vi "Start - Stop Postions1.vi"(5 "New Status of Positions":bool[](array[boolean]), 7 "Rack Number":i16=1 min=1 max=16, 11 "System#":u8=1 min=1 max=16) -> ()   [LabVIEW 2021]
uses:
  Main Controls System v8.0/AutoAge Globals.vi
panel:
  out "At least 1 position\nhas started":bool
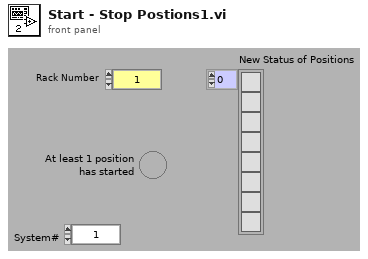
[diagram p1: front panel]
types:
  T1 = enum32{"existing file", "new file", "new or existing file", "existing dir", "new dir", "new or existing dir", "existing file (use LLBs)", "new file (use LLBs)", "new or existing file (use LLBs)", "new or existing file or directory (use LLBs)"}
  T2 = enum16{"open", "replace", "create", "open or create", "replace or create", "replace or create with confirmation"}
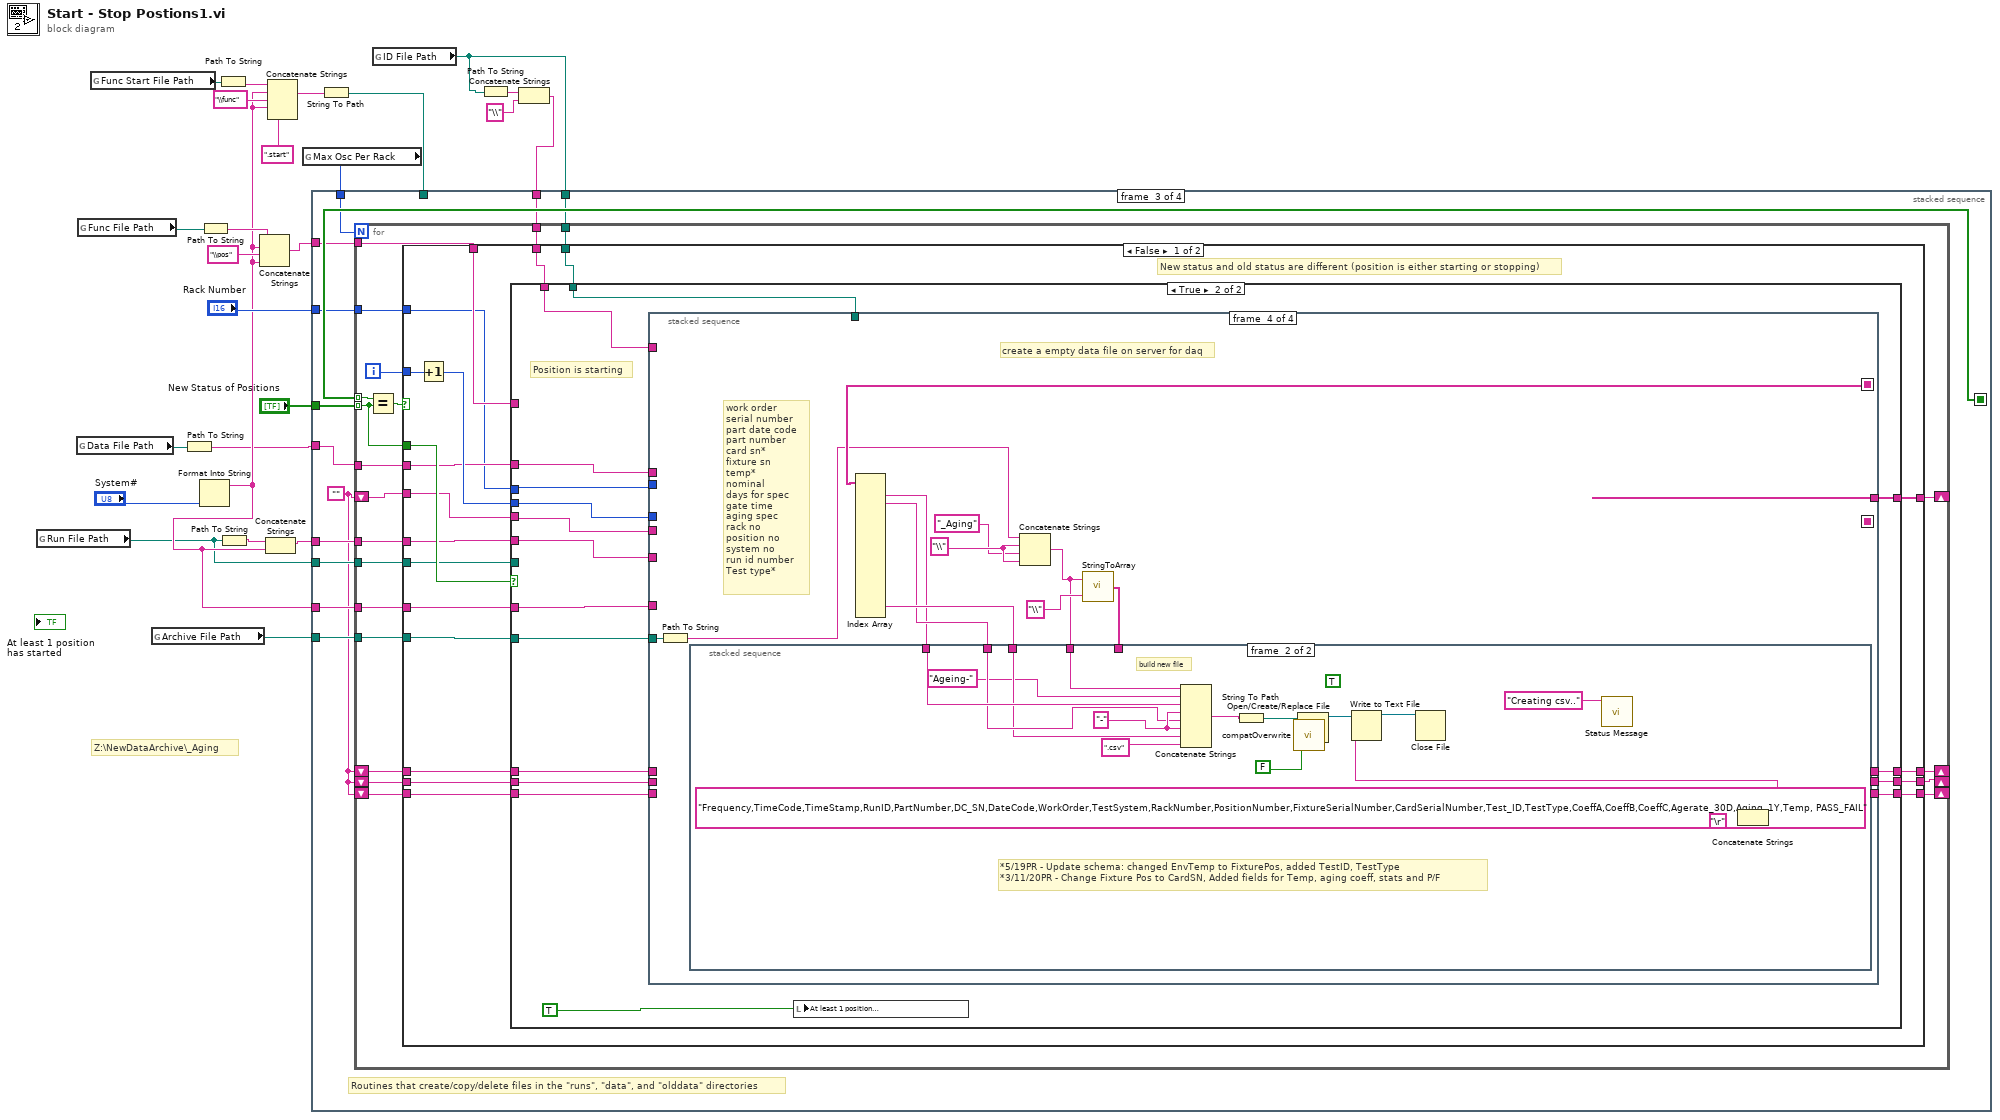
[diagram p0: block diagram]
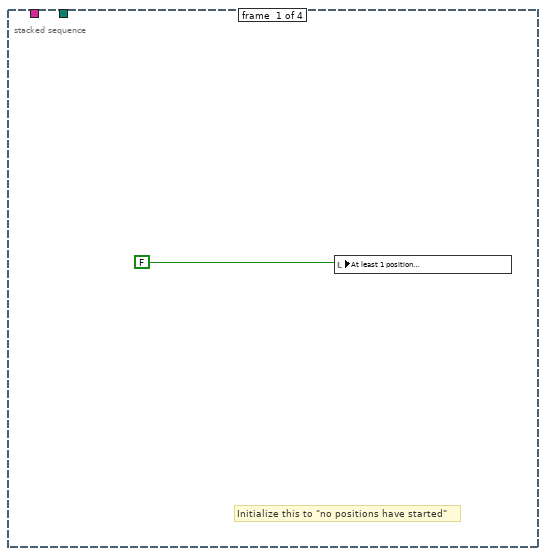
[diagram p2: hidden frame]
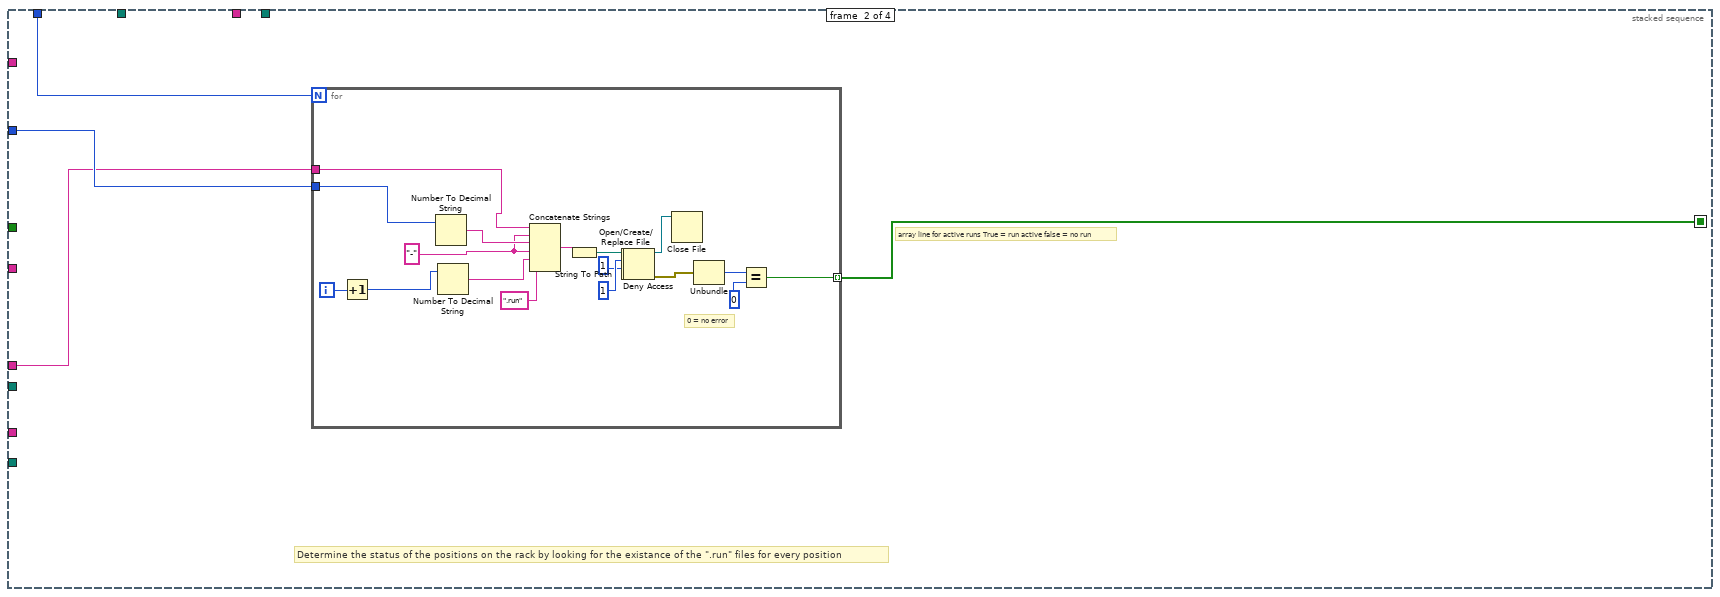
[diagram p3: hidden frame]
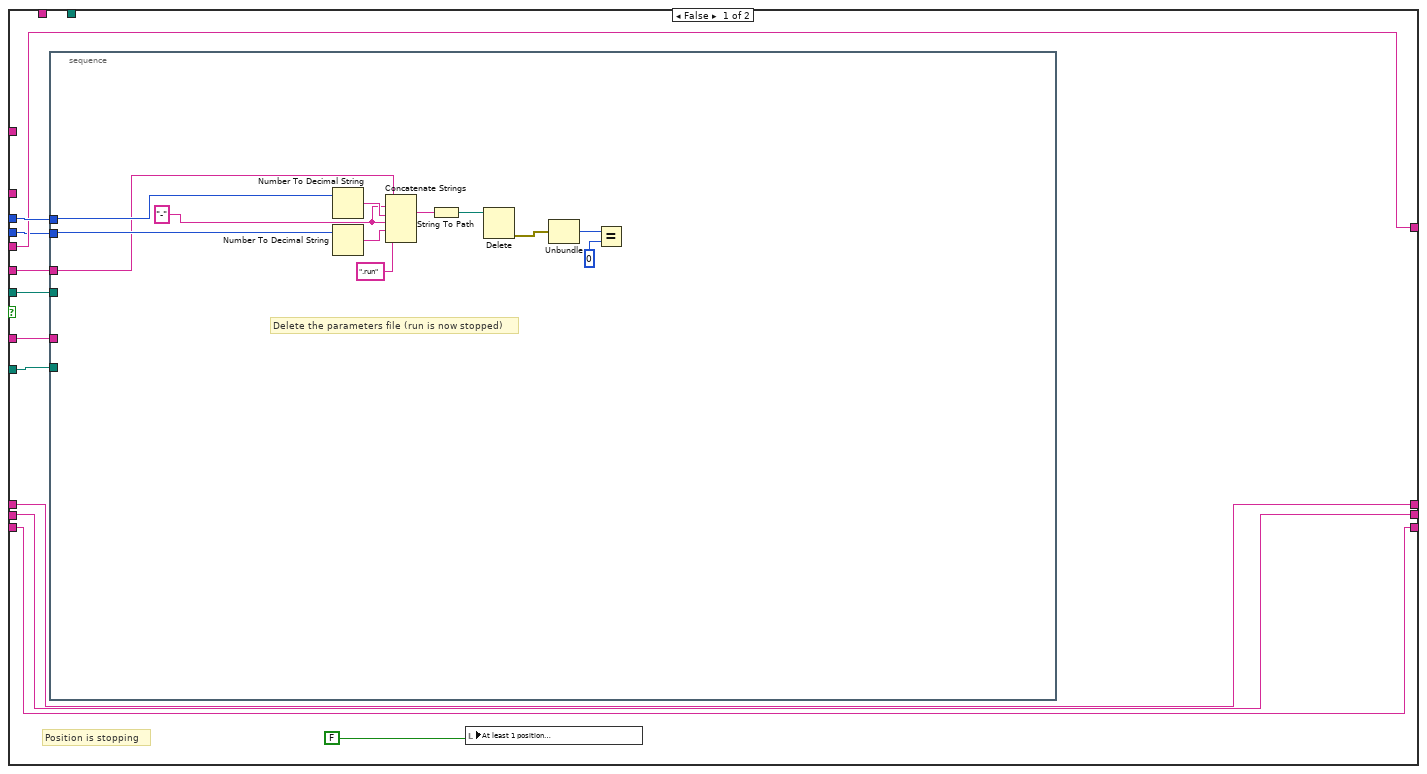
[diagram p4: hidden frame]
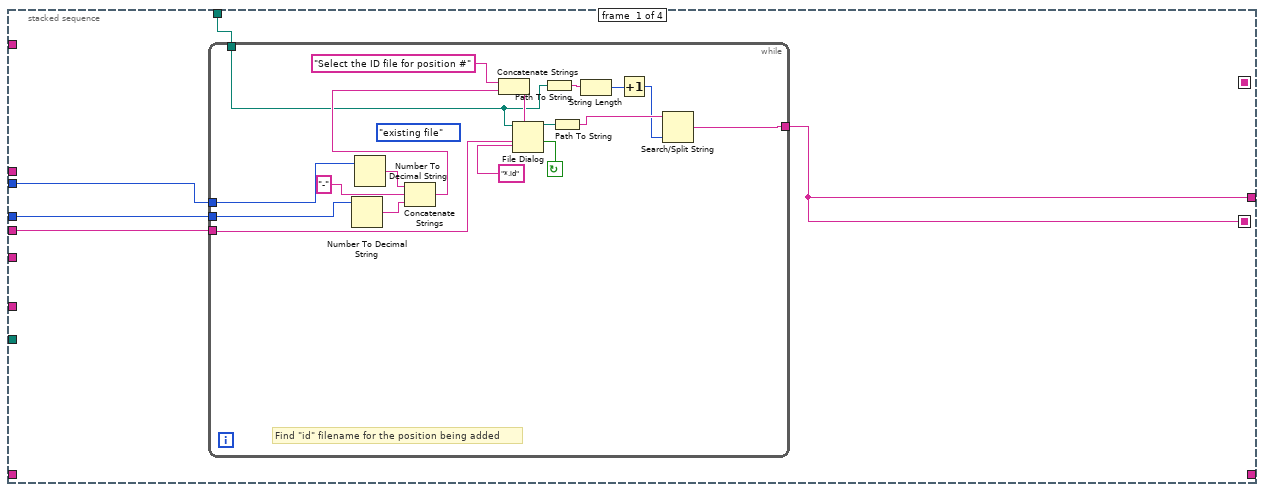
[diagram p5: hidden frame]
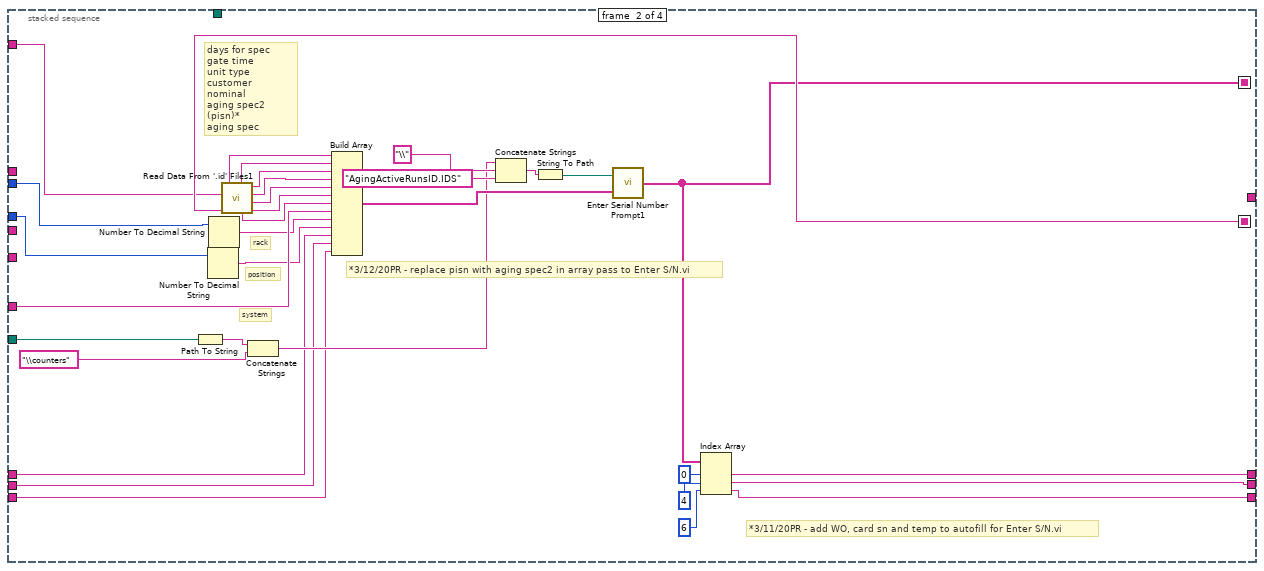
[diagram p6: hidden frame]
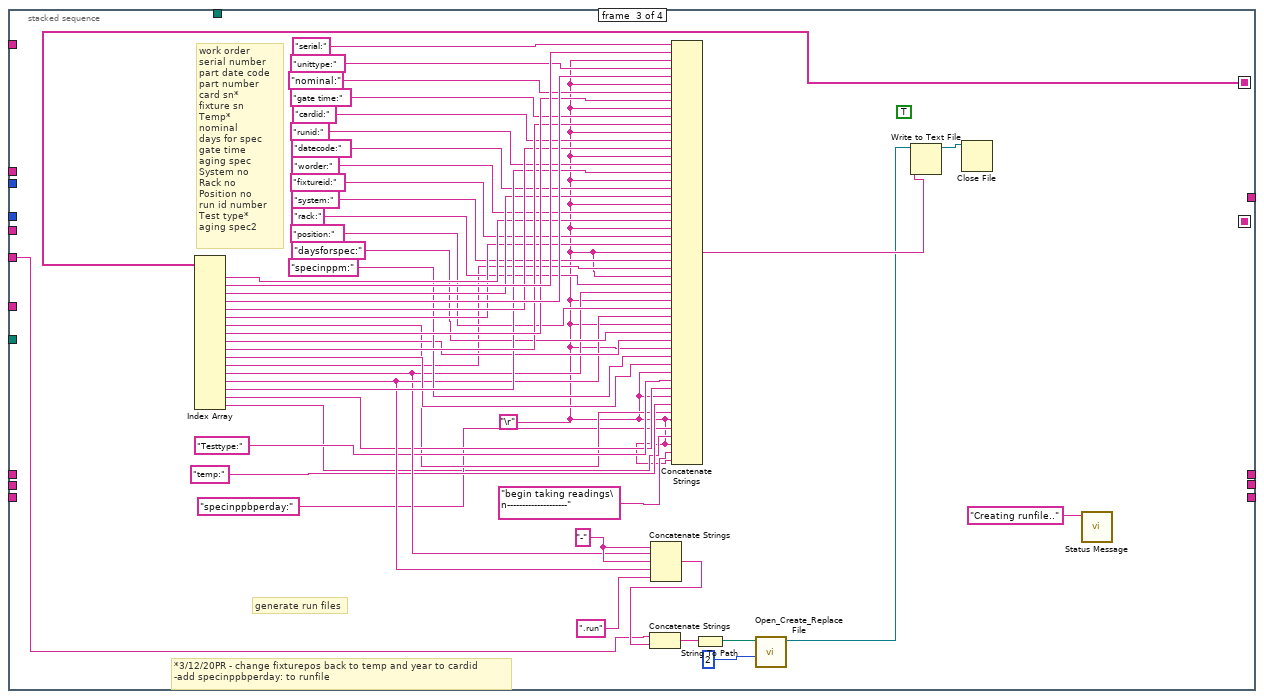
[diagram p7: hidden frame]
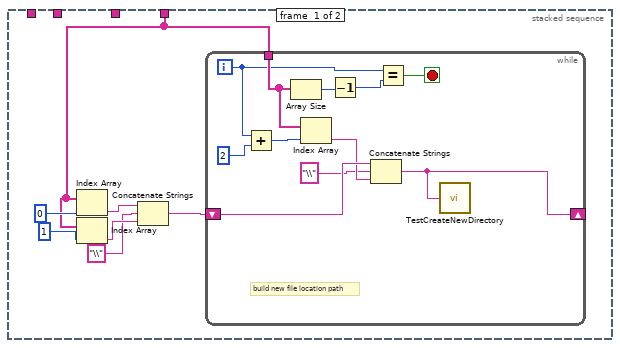
[diagram p8: hidden frame]
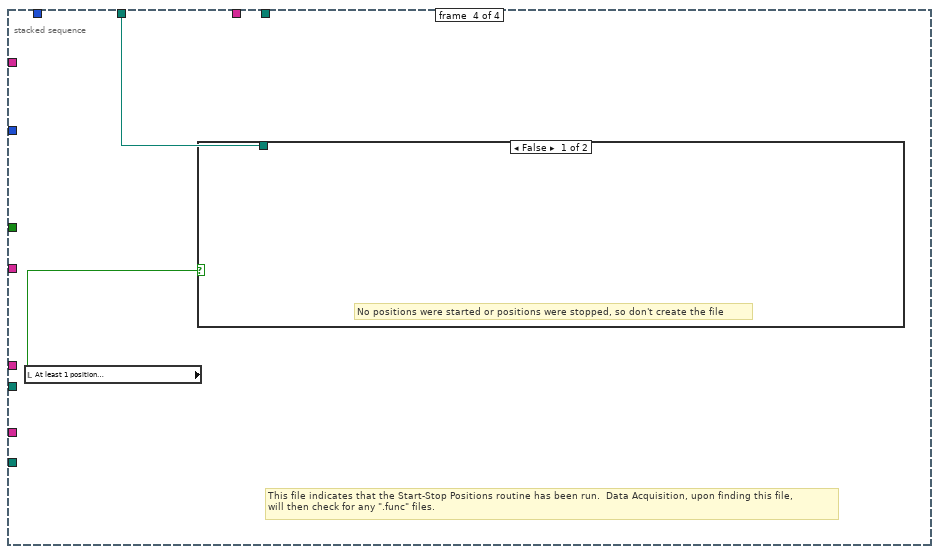
[diagram p10: hidden frame]
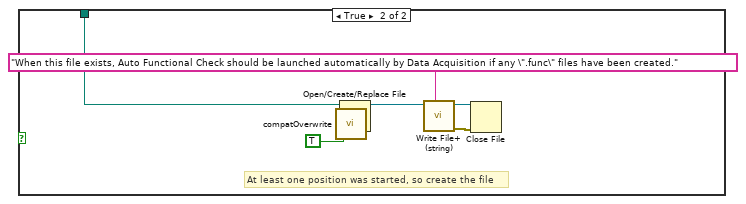
[diagram p11: hidden frame]
diagram:
  # "Z:\\NewDataArchive\\_Aging"
  n1 = global read "AutoAge Globals.vi" "Run File Path"() -> (w2:path)
  n2 = global read "AutoAge Globals.vi" "Data File Path"() -> (w15:path)
  n3 = global read "AutoAge Globals.vi" "Func File Path"() -> (w16:path)
  n4 = global read "AutoAge Globals.vi" "Func Start File Path"() -> (w17:path)
  n5 = global read "AutoAge Globals.vi" "Archive File Path"() -> (w14:path)
  n6 = Path To String(path=w15) -> (string=w1:string)
  n7 = Format Into String("System#") -> (resulting string=w3:string)  [unwired: 3 in, 1 out]
  n8 = Path To String(path=w16) -> (string=w21:string)
  n9 = Path To String(path=w17) -> (string=w8:string)
  n10 = Path To String(path=w2) -> (string=w22:string)
  n11 = Concatenate Strings(w21, w3, "\\pos" ("Substring"), w3) -> (w20:string)
  n12 = Concatenate Strings(w22, w3) -> (w23:string)
  n13 = Concatenate Strings(w8, w3, "\\func" ("Substring"), w3, ".start" ("Substring")) -> (w19:string)
  n14 = global read "AutoAge Globals.vi" "Max Osc Per Rack"() -> (w4:u16)
  n15 = String To Path(string=w19) -> (path=w18:path)
  n16 = global read "AutoAge Globals.vi" "ID File Path"() -> (w12:path)
  n17 = Path To String(path=w12) -> (string=w11:string)
  n18 = Concatenate Strings(w11, "\\" ("Substring")) -> (w9:string)
  n19 = stacked-sequence {
    seq-local: [_ w29 _ _] -> [_ _ w62 _]
    tunnel: "Rack Number" -> [_ w30 w54 _]
    tunnel: "New Status of Positions" -> [_ _ w61 _]
    tunnel: w9 -> [_ _ w59 _]
    tunnel: w23 -> [_ w27 w57 _]
    tunnel: w1 -> [_ _ w58 _]
    tunnel: w14 -> [_ _ w56 _]
    tunnel: w20 -> [_ _ w55 _]
    tunnel: w18 -> [_ _ _ w298]
    tunnel: w12 -> [_ _ w53 _]
    tunnel: w4 -> [_ w28 w60 _]
    tunnel: w3 -> [_ _ w52 _]
    tunnel: w2 -> [_ _ w51 _]
    frame #0 {
      # "Initialize this to \"no positions have started\""
      n20 = local write "At least 1 position\nhas started"(FALSE) -> ()
    }
    frame #1 {
      # "array line for active runs True = run active false = no run"
      # "Determine the status of the positions on the rack by looking for the existance of the \".run\" files for every position"
      n21 = for {
        N: w28 -> [_]
        tunnel: [w48] -> w29 mode=indexing
        tunnel: w30 -> [w38]
        tunnel: w27 -> [w33]
        i -> [w49]
        w34 = "-"
        # "0 = no error"
        n22 = Increment(x=w49) -> (x+1=w35:i32)
        n23 = Number To Decimal String(number=w38) -> (decimal integer string=w37:string)  [unwired: 1 in]
        n24 = Number To Decimal String(number=w35) -> (decimal integer string=w36:string)  [unwired: 1 in]
        n25 = Concatenate Strings(w33, w34, w37, w34, w36, ".run") -> (w47:string)
        n26 = String To Path(string=w47) -> (path=w46:path)
        n27 = Open/Create/Replace File(file path (use dialog)=w46, access (0:read/write)=1) -> (refnum out=w31:refnum<file>, error out=w32:errorcluster)  [unwired: 4 in, 1 out]
        n28 = Deny Access(4:w32, 6:1, 7:w31) -> (0:w43:errorcluster, 3:w40:refnum<file>)
        n29 = Close File(refnum=w40) -> ()  [unwired: 1 in, 2 out]
        n30 = Unbundle(w43) -> ("code"=w41:i32)  [unwired: 2 out]
        n31 = Equal?(x=w41, y=0) -> (x = y?=w48:bool)
      }
    }
    frame #2 {
      w50 = ""
      # "Routines that create/copy/delete files in the \"runs\", \"data\", and \"olddata\" directories"
      n32 = for {
        N: w60 -> [_]
        tunnel: w62 -> [w82] mode=indexing
        tunnel: w61 -> [w81] mode=indexing
        shift-right: [w78] -> _
        shift-left: w50 -> [w79]
        tunnel: w59 -> [w77]
        tunnel: w58 -> [w76]
        tunnel: w57 -> [w75]
        tunnel: w56 -> [w74]
        tunnel: w55 -> [w73]
        tunnel: w54 -> [w72]
        tunnel: w53 -> [w71]
        tunnel: w52 -> [w70]
        tunnel: w51 -> [w69]
        shift-right: [w68] -> _
        shift-left: w50 -> [w65]
        shift-right: [w67] -> _
        shift-left: w50 -> [w64]
        shift-right: [w66] -> _
        shift-left: w50 -> [w63]
        i -> [w80]
        n33 = Equal?(x=w82, y=w81) -> (x = y?=w83:bool)
        n34 = case shown="False" w83 {
          tunnel: w81 -> [w103 _]
          tunnel: w80 -> [w100 _]
          tunnel: w79 -> [w102 w297]
          tunnel: [w101 w297] -> w78
          tunnel: w77 -> [w98 _]
          tunnel: w76 -> [w97 _]
          tunnel: w75 -> [w96 _]
          tunnel: w74 -> [w95 _]
          tunnel: w73 -> [w94 _]
          tunnel: w72 -> [w93 _]
          tunnel: w71 -> [w92 _]
          tunnel: w70 -> [w91 _]
          tunnel: w69 -> [w90 _]
          tunnel: [w89 w296] -> w68
          tunnel: [w88 w295] -> w67
          tunnel: [w87 w294] -> w66
          tunnel: w65 -> [w86 w296]
          tunnel: w64 -> [w85 w295]
          tunnel: w63 -> [w84 w294]
          frame False {
            # "New status and old status are different (position is either starting or stopping)"
            n35 = Increment(x=w100) -> (x+1=w99:i32)
            n36 = case shown="True" w103 {
              tunnel: w93 -> [w114 w136]
              tunnel: w102 -> [w113 w143]
              tunnel: [w113 w142] -> w101
              tunnel: w99 -> [w112 w141]
              tunnel: w98 -> [_ w139]
              tunnel: w97 -> [_ w138]
              tunnel: w96 -> [w110 w137]
              tunnel: w95 -> [w109 w133]
              tunnel: w94 -> [_ _]
              tunnel: w92 -> [_ w135]
              tunnel: w91 -> [w108 w134]
              tunnel: w90 -> [w107 _]
              tunnel: [w106 w132] -> w89
              tunnel: [w105 w131] -> w88
              tunnel: [w104 w130] -> w87
              tunnel: w86 -> [w106 w129]
              tunnel: w85 -> [w105 w128]
              tunnel: w84 -> [w104 w127]
              frame False {
                # "Position is stopping"
                n37 = stacked-sequence {
                  tunnel: w114 -> [w118]
                  tunnel: w112 -> [w117]
                  tunnel: w110 -> [w115]
                  tunnel: w109 -> [_]
                  tunnel: w108 -> [_]
                  tunnel: w107 -> [_]
                  frame #0 {
                    w116 = "-"
                    # "Delete the parameters file (run is now stopped)"
                    n38 = Number To Decimal String(number=w118) -> (decimal integer string=w120:string)  [unwired: 1 in]
                    n39 = Number To Decimal String(number=w117) -> (decimal integer string=w119:string)  [unwired: 1 in]
                    n40 = Concatenate Strings(w115, w116, w120, w116, w119, ".run") -> (w126:string)
                    n41 = String To Path(string=w126) -> (path=w125:path)
                    n42 = Delete(path (use dialog)=w125) -> (error out=w123:errorcluster)  [unwired: 4 in, 2 out]
                    n43 = Unbundle(w123) -> ("code"=w124:i32)  [unwired: 2 out]
                    n44 = Equal?(x=w124, y=0) -> ()  [unwired: 1 out]
                  }
                }
                n45 = local write "At least 1 position\nhas started"(FALSE) -> ()
              }
              frame True {
                # "Position is starting"
                n46 = stacked-sequence {
                  seq-local: [w147 _ _ _] -> [_ w199 _ _]
                  seq-local: [_ w177 _ _] -> [_ _ w244 w258]
                  tunnel: w136 -> [w145 w190 _ _]
                  tunnel: w143 -> [w148 _ _ _]
                  tunnel: [w147 _ _ _] -> w142
                  tunnel: w141 -> [w146 w189 _ _]
                  tunnel: w139 -> [_ w198 _ _]
                  tunnel: w138 -> [_ _ _ _]
                  tunnel: w137 -> [_ _ w242 _]
                  tunnel: w135 -> [w144 _ _ _]
                  tunnel: w134 -> [_ w184 _ _]
                  tunnel: w133 -> [_ w181 _ w257]
                  tunnel: [_ w173 _ _] -> w132
                  tunnel: [_ w172 _ _] -> w131
                  tunnel: [_ w171 _ _] -> w130
                  tunnel: w129 -> [_ w170 _ _]
                  tunnel: w128 -> [_ w169 _ _]
                  tunnel: w127 -> [_ w168 _ _]
                  frame #0 {
                    n47 = while {
                      tunnel: w144 -> [w153]
                      tunnel: w146 -> [w158]
                      tunnel: w145 -> [w156]
                      tunnel: [w149] -> w147
                      tunnel: w148 -> [w165]
                      stop <- w166 continue-if-true
                      (unwired) T1."existing file" ("select mode (2)")
                      # "Find \"id\" filename for the position being added"
                      n48 = Number To Decimal String(number=w158) -> (decimal integer string=w160:string)  [unwired: 1 in]
                      n49 = Number To Decimal String(number=w156) -> (decimal integer string=w155:string)  [unwired: 1 in]
                      n50 = Concatenate Strings(w155, "-", w160) -> (w157:string)
                      n51 = Concatenate Strings("Select the ID file for position #" ("prompt"), w157) -> (w161:string)
                      n52 = File Dialog(6:"*.id" ("pattern"), 7:w161, 9:w165, 11:w153) -> (1:w166:bool, 3:w163:path)  [unwired: 3 in, 2 out]
                      n53 = Path To String(path=w153) -> (string=w152:string)
                      n54 = Path To String(path=w163) -> (string=w162:string)
                      n55 = String Length(string=w152) -> (length=w151:i32)
                      n56 = Increment(x=w151) -> (x+1=w150:i32)
                      n57 = Search/Split String(string=w162, offset (0)=w150) -> (match + rest of string=w149:string)  [unwired: 1 in, 2 out]
                    }
                  }
                  frame #1 {
                    # "*3/12/20PR - replace pisn with aging spec2 in array pass to Enter S/N.vi"
                    # "*3/11/20PR - add WO, card sn and temp to autofill for Enter S/N.vi"
                    # "system"
                    # "position"
                    # "rack"
                    # "days for spec\ngate time\nunit type\ncustomer\nnominal\naging spec2 (pisn)*\naging spec"
                    n58 = Path To String(path=w181) -> (string=w180:string)
                    n59 = Number To Decimal String(number=w189) -> (decimal integer string=w182:string)  [unwired: 1 in]
                    n60 = Number To Decimal String(number=w190) -> (decimal integer string=w183:string)  [unwired: 1 in]
                    n61 = call "Read Data From '.id' Files1.vi"("ID File Path"=w198, "ID Filename"=w199) -> ("# Days for Aging Spec"=w197:string, "Gate Time"=w196:string, "Aging Spec"=w192:string, "Unit Type"=w195:string, "Customer"=w194:string, "Nominal Frequency"=w193:string, "Aging Spec 2"=w167:string)  [unwired: 1 out]
                    n62 = Concatenate Strings(w180, "\\counters") -> (w178:string)
                    n63 = Build Array(w197, w196, w195, w194, w193, w167, w192, w184, w183, w182, w170, w169, w168) -> (w191:string[])
                    n64 = Concatenate Strings(w178, "\\", "AgingActiveRunsID.IDS") -> (w185:string)
                    n65 = String To Path(string=w185) -> (path=w188:path)
                    n66 = call "Enter Serial Number Prompt1.vi"("InputArray"=w191, "data storage path"=w188) -> ("OutputArray"=w177:string[])
                    n67 = Index Array(array=w177, index #1=0 ("index"), index #2=4 ("index"), index #3=6 ("index")) -> (element #1=w173:string, element #2=w172:string, element #3=w171:string)
                  }
                  frame #2 {
                    (unwired) TRUE
                    w201 = "\r"
                    w218 = "-"
                    # "*3/12/20PR - change fixturepos back to temp and year to cardid\n-add specinppbperday: to runfile"
                    # "work order\nserial number\npart date code\npart number\ncard sn*\nfixture sn\nTemp*\nnominal\ndays for spec\ngate time\naging spec\nSystem no\nRack no\nPosition no\nrun id number\nTest type*\naging spec2"
                    # "generate run files"
                    n68 = Index Array(array=w244) -> (element #1=w226:string, element #2=w240:string, element #3=w228:string, element #4=w238:string, element #5=w232:string, element #6=w224:string, element #7=w205:string, element #8=w236:string, element #9=w215:string, element #10=w234:string, element #11=w217:string, element #12=w209:string, element #13=w211:string, element #14=w213:string, element #15=w230:string, element #16=w207:string, element #17=w203:string)  [unwired: 17 in]
                    n69 = Concatenate Strings(w218, w211, w218, w213, ".run") -> (w243:string)
                    n70 = Concatenate Strings(w242, w243) -> (w246:string)
                    n71 = Concatenate Strings("serial:", w240, w201, "unittype:", w238, w201, "nominal:", w236, w201, "gate time:", w234, w201, "cardid:", w232, w201, "runid:", w230, w201, "datecode:", w228, w201, "worder:", w226, w201, "fixtureid:", w224, w201, "system:", w209, w201, "rack:", w211, w201, "position:", w213, w201, "daysforspec:", w215, w201, "specinppm:", w217, w201, "Testtype:", w207, w201, "temp:", w205, w201, "specinppbperday:" ("string"), w203, w201, "begin taking readings\n--------------------", w201) -> (w222:string)
                    n72 = String To Path(string=w246) -> (path=w220:path)
                    n73 = call <vilib>:"Open_Create_Replace File.vi"("function (open:0)"=2, "file path"=w220) -> ("refnum"=w219:refnum<file>)  [unwired: 6 in, 3 out]
                    n74 = Write to Text File(file (use dialog)=w219, text=w222) -> (refnum out=w221:refnum<file>)  [unwired: 2 in, 2 out]
                    n75 = Close File(refnum=w221) -> ()  [unwired: 1 in, 2 out]
                    n76 = call "Status Message.vi"(11:"Creating runfile..") -> ()  [unwired: 11 in]
                  }
                  frame #3 {
                    w253 = "\\"
                    # "work order\nserial number\npart date code\npart number\ncard sn*\nfixture sn\ntemp*\nnominal\ndays for spec\ngate time\naging spec\nrack no\nposition no\nsystem no\nrun id number\nTest type*"
                    # "create a empty data file on server for daq"
                    n77 = Path To String(path=w257) -> (string=w256:string)
                    n78 = Index Array(array=w258) -> (element #1=w249:string, element #2=w250:string, element #15=w251:string)  [unwired: 16 in, 13 out]
                    n79 = Concatenate Strings(w256, w253, "_Aging", w253) -> (w252:string)
                    n80 = call "StringToArray.vi"("String Delimiter"="\\", "Input String"=w252) -> ("Array"=w254:string[])
                    n81 = stacked-sequence {
                      tunnel: w254 -> [w260 _]
                      tunnel: w252 -> [_ w280]
                      tunnel: w251 -> [_ w281]
                      tunnel: w250 -> [_ w282]
                      tunnel: w249 -> [_ w285]
                      frame #0 {
                        n82 = Index Array(array=w260, index=0) -> (element=w263:string)
                        n83 = Index Array(array=w260, index=1) -> (element=w265:string)
                        n84 = Concatenate Strings(w263, "\\", w265) -> (w259:string)
                        n85 = while {
                          tunnel: w260 -> [w275]
                          shift-right: [w266] -> _
                          shift-left: w259 -> [w273]
                          i -> [w269]
                          stop <- w270 stop-if-true
                          # "build new file location path"
                          n86 = Add(x=w269, y=2) -> (x+y=w274:i32)
                          n87 = Array Size(array=w275) -> (size(s)=w268:i32)
                          n88 = Index Array(array=w275, index=w274) -> (element=w272:string)
                          n89 = Decrement(x=w268) -> (x-1=w267:i32)
                          n90 = Concatenate Strings(w273, "\\", w272) -> (w266:string)
                          n91 = Equal?(x=w269, y=w267) -> (x = y?=w270:bool)
                          n92 = call "TestCreateNewDirectory.vi"("NewDirectory"=w266) -> ()  [unwired: 1 out]
                        }
                      }
                      frame #1 {
                        (unwired) TRUE
                        w283 = "-"
                        # "*5/19PR - Update schema: changed EnvTemp to FixturePos, added TestID, TestType \n*3/11/20PR - Change Fixture Pos to CardSN, Added fields for Temp, aging coeff, stats and P/F"
                        # "build new file"
                        n93 = Concatenate Strings(w280, "Ageing-", w285, w283, w282, w283, w281, ".csv") -> (w293:string)
                        n94 = String To Path(string=w293) -> (path=w292:path)
                        n95 = call <vilib>:"compatOverwrite.vi"("overwrite (F)"=FALSE) -> ("overwrite?"=w278:T2)
                        n96 = Open/Create/Replace File(file path (use dialog)=w292, operation (0:open)=w278) -> (refnum out=w290:refnum<file>)  [unwired: 4 in, 2 out]
                        n97 = call "Status Message.vi"(11:"Creating csv..") -> ()  [unwired: 11 in]
                        n98 = Concatenate Strings("Frequency,TimeCode,TimeStamp,RunID,PartNumber,DC_SN,DateCode,WorkOrder,TestSystem,RackNumber,PositionNumber,FixtureSerialNumber,CardSerialNumber,Test_ID,TestType,CoeffA,CoeffB,CoeffC,Agerate_30D,Aging_1Y,Temp, PASS_FAIL", "\r") -> (w286:string)
                        n99 = Write to Text File(file (use dialog)=w290, text=w286) -> (refnum out=w289:refnum<file>)  [unwired: 2 in, 2 out]
                        n100 = Close File(refnum=w289) -> ()  [unwired: 1 in, 2 out]
                      }
                    }
                  }
                }
                n101 = local write "At least 1 position\nhas started"(TRUE) -> ()
              }
            }
          }
          frame True {
            # "New status and old status are the same, no changes need to be made"
          }
        }
      }
    }
    frame #3 {
      # "This file indicates that the Start-Stop Positions routine has been run.  Data Acquisition, upon finding this file, \nwill then check for any \".func\" files."
      n102 = local read "At least 1 position\nhas started"() -> (w299:bool)
      n103 = case shown="False" w299 {
        tunnel: w298 -> [_ w301]
        frame False {
          # "No positions were started or positions were stopped, so don't create the file"
        }
        frame True {
          # "At least one position was started, so create the file"
          n104 = call <vilib>:"compatOverwrite.vi"("overwrite (F)"=TRUE) -> ("overwrite?"=w300:T2)
          n105 = Open/Create/Replace File(file path (use dialog)=w301, operation (0:open)=w300) -> (refnum out=w303:refnum<file>)  [unwired: 4 in, 2 out]
          n106 = call <vilib>:"Write File+ (string).vi"("string"="When this file exists, Auto Functional Check should be launched automatically by Data Acquisition if any \".func\" files have been created.", "refnum"=w303) -> ("error out"=w305:errorcluster, "dup refnum"=w306:refnum<file>)  [unwired: 5 in, 1 out]
          n107 = Close File(refnum=w306, error in=w305) -> ()  [unwired: 2 out]
        }
      }
    }
  }
